vi "Receiver_Example - 2 Channel - Experiment_4.vi"() -> ()   [LabVIEW 2022 SP3]
panel:
  in  "Counter":dbl
  in  "State":i32
  out "CH0":bool
  out "CH1":bool
  out "iterationsIM":dbl
  out "High-Power Image 2":T1(plugin-control)
  out "High-Power Decoded message - CH0":string
  out "High-Power BER":T2(graph)
  in  "High-Power Window Size":dbl=15.0 format="%#_6p"
  in  "Low-Power Window Size - CH0":dbl=15.0 format="%#_6p"
  out "Low-Power BER - CH0":dbl(graph)
  out "Constellation Map":cluster{"Constellation":cdb[]}[](graph)
  in  "Tab Control":enum32{"USRP Parameters", "Rx Info", "BER"}(tab)
  in  "USRP ControledParameters":T3={"Active Antenna"="RX2", "Gain (dB)"=10.0, "Carrier Frequency"=2400000000.0, "IQ Rate"=2000000.0, "Active channels"="0,1"} {"IQ Rate" format="%#_6p"; "Carrier Frequency" format="%#_6p"; "Gain (dB)" format="%#_6f"}
  in  "Device selection":refnum<k15>="RIO0"
  in  "Trigger level":dbl=0.005 format="%f"
  out "CH0":T4
  out "CH1":T4
  out "SIG valid? - CH1":bool
  out "SIG valid? - CH0":bool
  out "Frequency offset - CH1":dbl
  out "Frequency offset - CH0":dbl
  out "Coerced Parameters":T5={"IQ Rate"=100000.0, "Carrier  Freq."=100000.0, "Gain"=0.0} {"Gain" format="%#_6f"; "Carrier  Freq." format="%#_6p"; "IQ Rate" format="%#_6p"}
  out "Error out":errorcluster
  in  "Expected message LP - CH0":string="Non Critical Data\nNon Critical Data\nNon Critical Data\nNon Critical Data\nNon Critical Data"
  in  "Expected message - CH1":string="Critical Dataaaaa\nCritical Dataaaaa\nCritical Dataaaaa\nCritical Dataaaaa\nCritical Dataaaaa"
  out "Expected message LP Detected CH0":string="Non Critical Data\nNon Critical Data\nNon Critical Data\nNon Critical Data\nNon Critical Data"
  out "Expected message HP Detected CH1":string="Non Critical Data\nNon Critical Data\nNon Critical Data\nNon Critical Data\nNon Critical Data"
  in  "Boolean":bool
  in  "Boolean 3":bool
  out "Expected message HP Detected CH0":string="Non Critical Data\nNon Critical Data\nNon Critical Data\nNon Critical Data\nNon Critical Data"
  in  "Expected message HP - CH0":string="Critical Dataaaaa\nCritical Dataaaaa\nCritical Dataaaaa\nCritical Dataaaaa\nCritical Dataaaaa"
  in  "Boolean 2":bool
  out "Inst. BER HP - CH0":dbl format="%#_4g"
  out "Acc. BER HP - CH0":dbl format="%#_4g"
  out "Acum. Err HP - CH0":dbl
  out "No. Bits HP - CH0":dbl
  out "Acc. BER LP - CH0":dbl format="%#_4g"
  out "Inst. BER - CH1":dbl format="%#_4g"
  out "Inst. BER LP - CH0":dbl format="%#_4g"
  out "No. Bits - CH1":dbl
  out "No. Bits LP - CH0":dbl
  out "Acum. Err - CH1":dbl
  out "Acum. Err LP - CH0":dbl
  in  "Record BER":bool
  in  "Refresh Button":bool
  out "Acc. BER - CH1":dbl format="%#_4g"
  in  "error in (no error)":errorcluster
  out "Decoded message - CH1":string
  out "Low-Power Decoded message - CH0":string
  # "OFDM Superposition Coded Receiver"
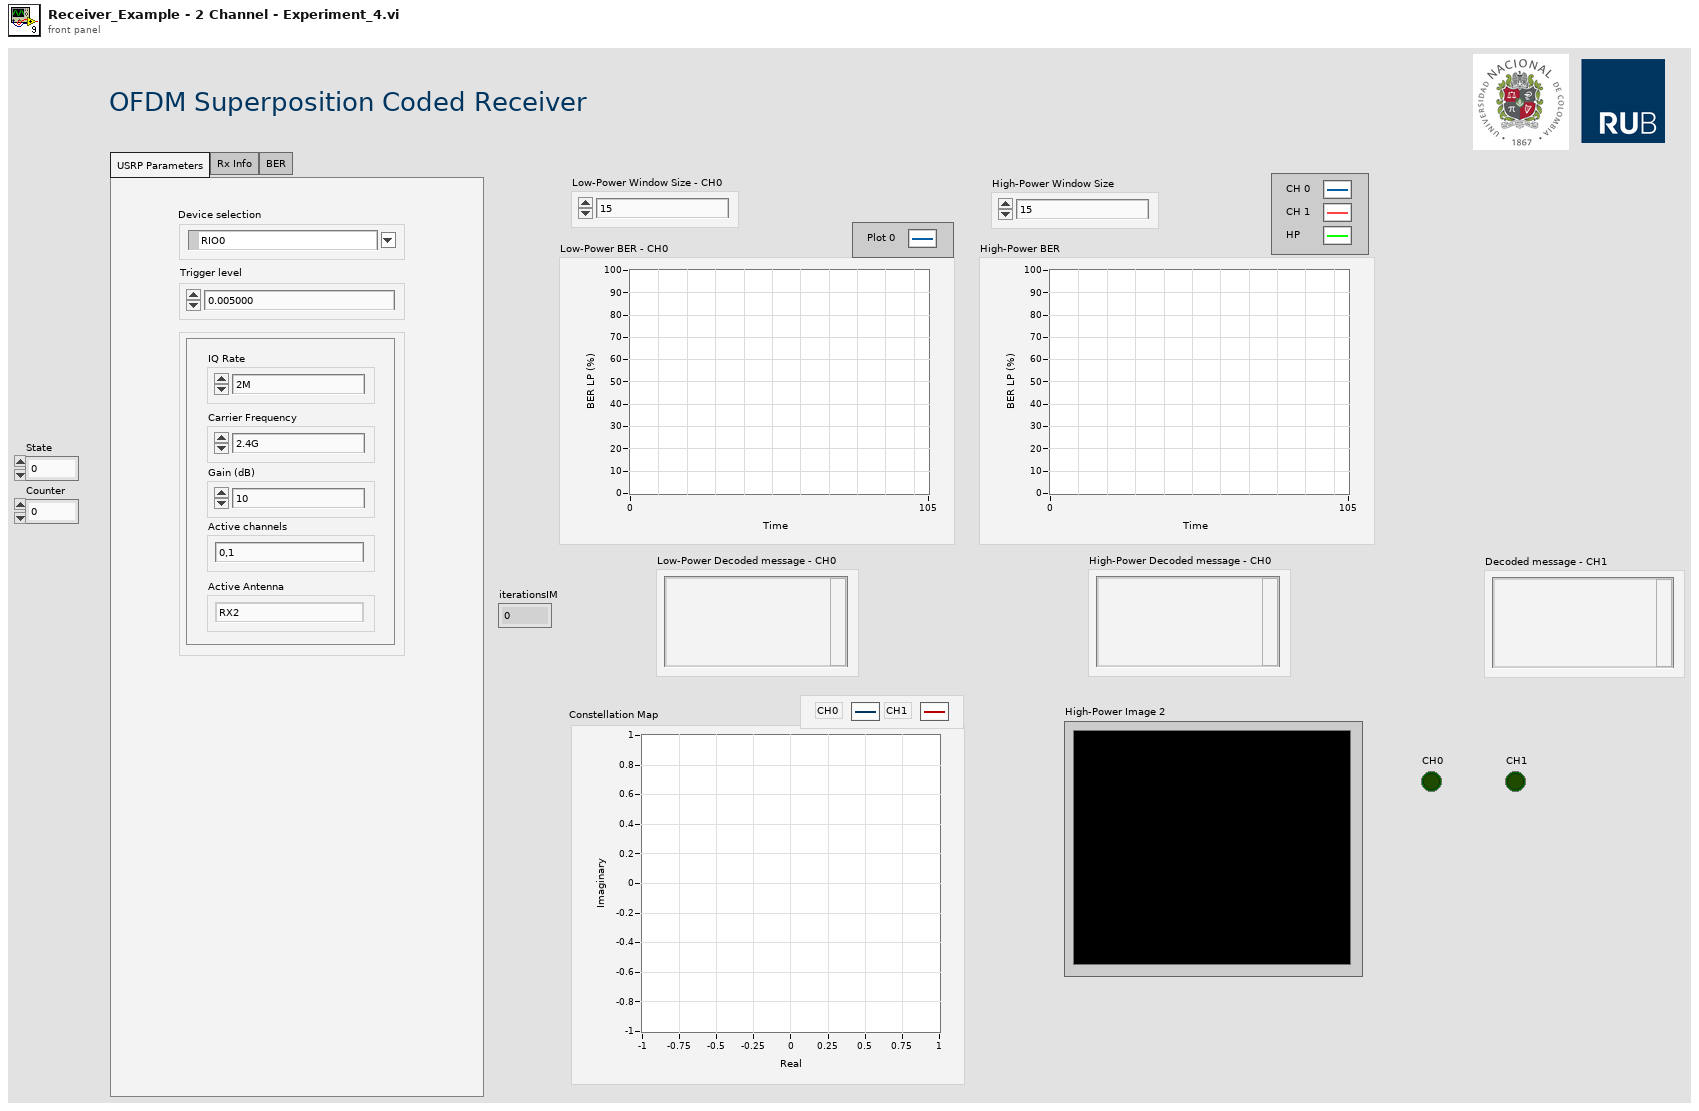
[diagram p1: front panel]
types:
  T1 = typedef "IMAQ Image.ctl" = refnum<image>
  T2 = cluster{"Graph Instantaneous BER":dbl, "Graph Instantaneous BER":dbl, "Inst. BER - CH1":dbl}
  T3 = cluster{"Active Antenna":string, "Gain (dB)":dbl, "Carrier Frequency":dbl, "IQ Rate":dbl, "Active channels":string}
  T4 = cluster{"Modulation type":enum16{"QPSK(4QAM)", "64QAM", "16QAM", "BPSK"}, "BCC rate (k/n)":enum16{"1/2", "2/3", "3/4"}}
  T5 = cluster{"IQ Rate":dbl, "Carrier  Freq.":dbl, "Gain":dbl}
  T6 = cluster{"coerced IQ rate":dbl, "coerced carrier frequency":dbl, "coerced gain":dbl}
  T7 = cluster{"Graph Instantaneous BER":dbl, "Graph Instantaneous BER":dbl, "Graph Instantaneous BER":dbl}
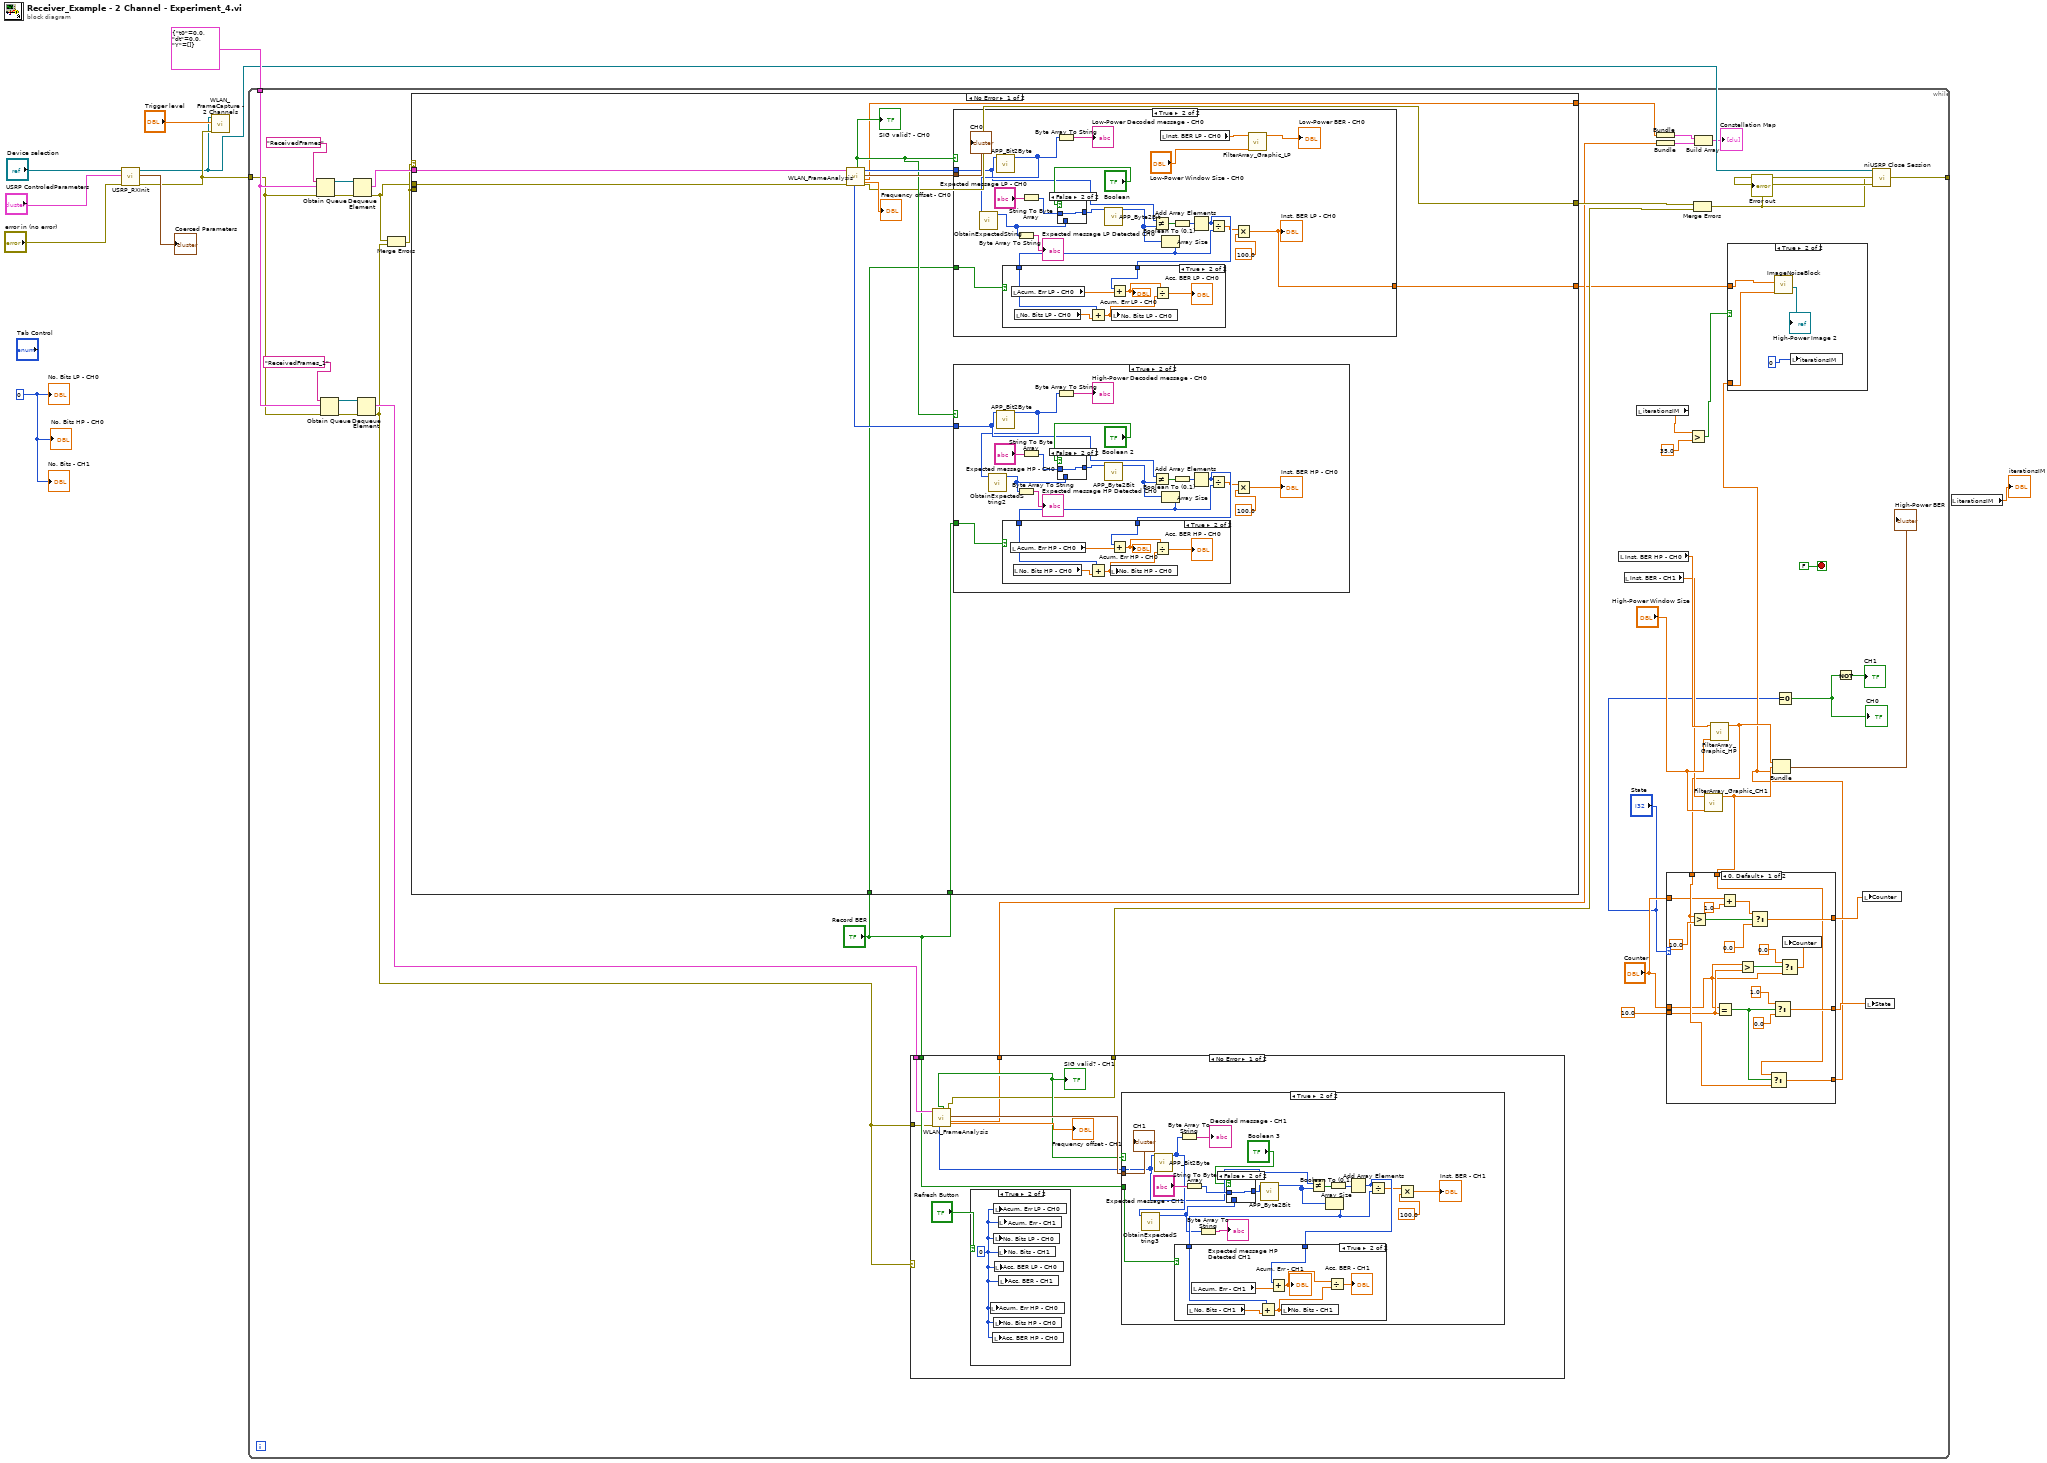
[diagram p0: block diagram]
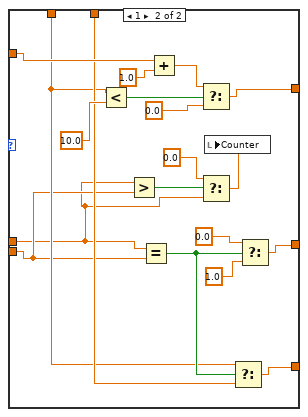
[diagram p2: hidden frame]
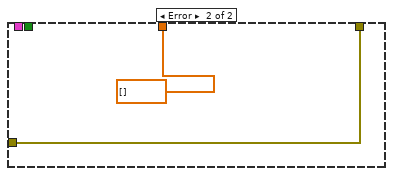
[diagram p7: hidden frame]
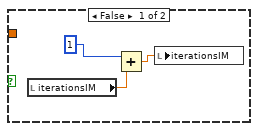
[diagram p8: hidden frame]
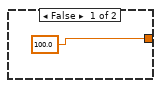
[diagram p12: hidden frame]
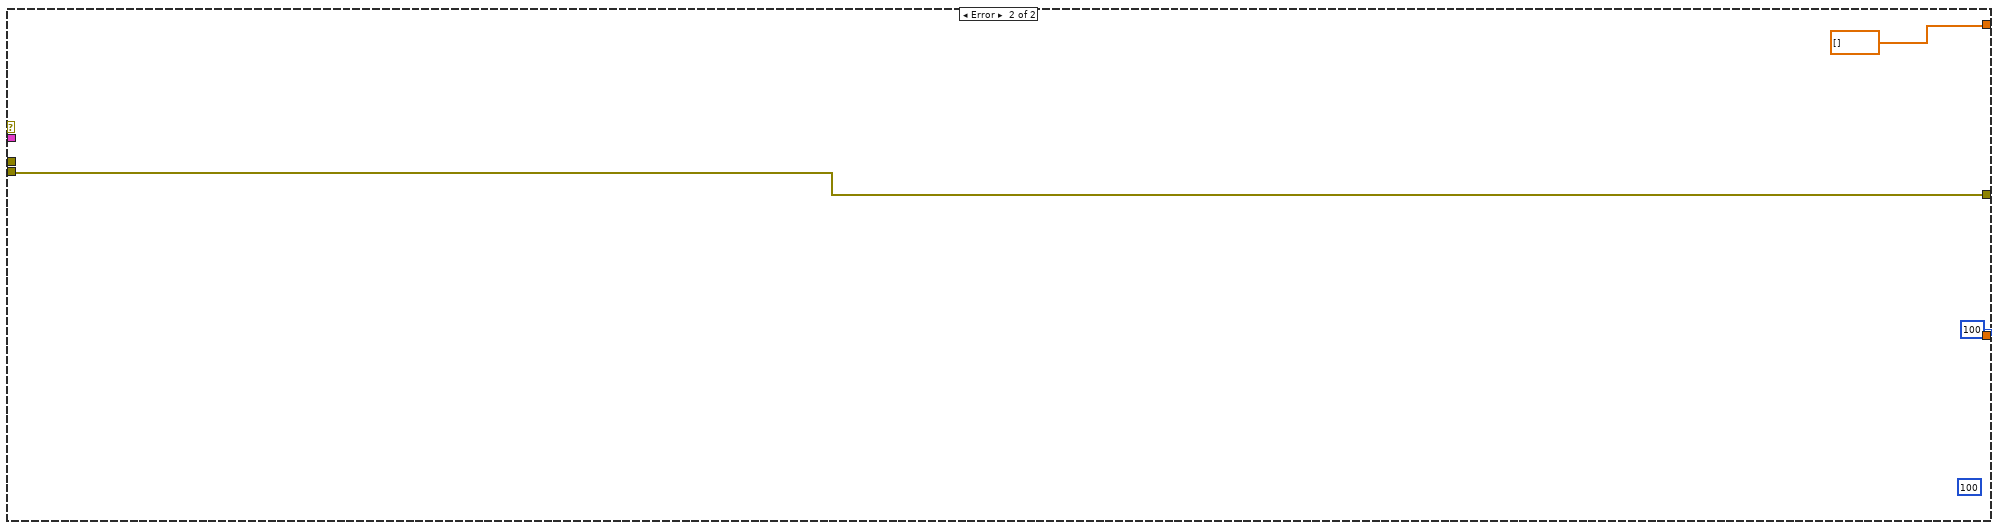
[diagram p15: hidden frame]
diagram:
  w2 = 0
  n1 = call "USRP_RXInit.vi"("device names"="Device selection", "USRP ControledParameters"="USRP ControledParameters", "error in (no error)"="error in (no error)") -> ("session handle out"=w5:refnum<k15>, "USRP CoercedParamters"=→"Coerced Parameters":T6, "error out"=w9:errorcluster)  [unwired: 5 in]
  n2 = call "WLAN_FrameCapture - 2 Channels.vi"("error in (no error)"=w9, "Trigger level"="Trigger level", "session handle"=w5) -> ()  [unwired: 8 in]
  n3 = while {
    tunnel: w9 -> [w44]
    tunnel: cluster{"t0":dbl, "dt":dbl, "Y":cdb[]} {"t0"=0.0, "dt"=0.0, "Y"=[]} ("data") -> [w45]
    tunnel: [w30] -> w6
    stop <- FALSE stop-if-true
    n4 = Obtain Queue(name (unnamed)="ReceivedFrames", element data type=w45, error in (no error)=w44) -> (queue out=w52:refnum<queue>, error out=w50:errorcluster)  [unwired: 2 in, 1 out]
    n5 = Obtain Queue(name (unnamed)="ReceivedFrames_1", element data type=w45, error in (no error)=w44) -> (queue out=w48:refnum<queue>, error out=w47:errorcluster)  [unwired: 2 in, 1 out]
    n6 = Dequeue Element(queue=w52, error in (no error)=w50) -> (element=w51:cluster{"t0":dbl, "dt":dbl, "Y":cdb[]}, error out=w41:errorcluster)  [unwired: 1 in, 2 out]
    n7 = Dequeue Element(queue=w48, error in (no error)=w47) -> (element=w33:cluster{"t0":dbl, "dt":dbl, "Y":cdb[]}, error out=w28:errorcluster)  [unwired: 1 in, 2 out]
    n8 = Merge Errors(w41, w28) -> (w42:errorcluster)
    n9 = case shown="No Error" w42 {
      tunnel: w51 -> [w147 _]
      tunnel: w42 -> [_ w211]
      tunnel: w41 -> [w144 _]
      tunnel: [w143 100] -> w26
      tunnel: [w142 dbl[] []] -> w34
      tunnel: [w141 w211] -> w32
      tunnel: "Record BER" -> [w140 _]
      tunnel: "Record BER" -> [w139 _]
      frame No Error {
        n10 = call "WLAN_FrameAnalysis.vi"("error in (no error)"=w144, "input cluster"=w147) -> ("error out"=w141:errorcluster, "Constellation"=w142:cdb[], "Modulation parameter"=w148:T4, "output bits"=w149:i8[], "Frequency offset"=→"Frequency offset - CH0":dbl, "SIG valid?"=w145:bool, "outputbitsHP"=w146:i8[])  [unwired: 3 in]
        "SIG valid? - CH0" <- w145
        n11 = case shown="True" w145 {
          tunnel: w149 -> [_ w181]
          tunnel: w148 -> [_ w199]
          tunnel: w139 -> [_ w195]
          tunnel: [100.0 w180] -> w143
          frame False {
          }
          frame True {
            n12 = call "APP_Bit2Byte.vi"("input bit stream"=w181) -> ("output byte stream"=w185:u8[])  [unwired: 10 in]
            n13 = call "ObtainExpectedString.vi"("Array"=w185) -> ("detectedMessage"=w182:i8[])  [unwired: 9 in]
            n14 = Byte Array To String(unsigned byte array=w182) -> (string=→"Expected message LP Detected CH0":string)
            n15 = String To Byte Array(string="Expected message LP - CH0") -> (unsigned byte array=w186:u8[])
            n16 = Byte Array To String(unsigned byte array=w185) -> (string=→"Low-Power Decoded message - CH0":string)
            n17 = case shown="False" "Boolean" {
              tunnel: [w201 w202] -> w188
              tunnel: w186 -> [_ w202]
              tunnel: w182 -> [w201 _]
              frame True {
              }
              frame False {
              }
            }
            n18 = call "APP_Byte2Bit.vi"("input byte stream"=w188) -> ("output bit stream"=w187:i8[])  [unwired: 10 in]
            n19 = Not Equal?(x=w181, y=w187) -> (x != y?=w197:bool[])
            n20 = local read "Inst. BER LP - CH0"() -> (w191:dbl)
            n21 = Array Size(array=w187) -> (size(s)=w194:i32)
            n22 = Boolean To (0,1)(Boolean=w197) -> (0, 1=w198:i16[])
            n23 = Add Array Elements(numeric array=w198) -> (sum=w193:i16)
            n24 = case shown="True" w195 {
              tunnel: w194 -> [_ w208]
              tunnel: w193 -> [_ w206]
              frame False {
              }
              frame True {
                n25 = local read "Acum. Err LP - CH0"() -> (w207:dbl)
                n26 = local read "No. Bits LP - CH0"() -> (w209:dbl)
                n27 = Add(x=w208, y=w209) -> (x+y=w205:dbl)
                n28 = Add(x=w206, y=w207) -> (x+y=w204:dbl)
                "Acum. Err LP - CH0" <- w204
                n29 = local write "No. Bits LP - CH0"(w205) -> ()
                n30 = Divide(x=w204, y=w205) -> (x/y=→"Acc. BER LP - CH0":dbl)
              }
            }
            n31 = Divide(x=w193, y=w194) -> (x/y=w190:dbl)
            n32 = Multiply(x=w190, y=100.0) -> (x*y=w180:dbl)
            "Inst. BER LP - CH0" <- w180
            n33 = call "FilterArray_Graphic_LP.vi"("Window Size"="Low-Power Window Size - CH0", "Instantaneous BER"=w191) -> ("Graph Instantaneous BER"=→"Low-Power BER - CH0":dbl)  [unwired: 4 in, 1 out]
            "CH0" <- w199
          }
        }
        n34 = case shown="True" w145 {
          tunnel: w146 -> [_ w154]
          tunnel: w140 -> [_ w164]
          frame False {
          }
          frame True {
            n35 = call "APP_Bit2Byte.vi"("input bit stream"=w154) -> ("output byte stream"=w153:u8[])  [unwired: 10 in]
            n36 = call "ObtainExpectedString2.vi"("Array"=w153) -> ("detectedMessage"=w152:i8[])  [unwired: 9 in]
            n37 = Byte Array To String(unsigned byte array=w152) -> (string=→"Expected message HP Detected CH0":string)
            n38 = String To Byte Array(string="Expected message HP - CH0") -> (unsigned byte array=w157:u8[])
            n39 = Byte Array To String(unsigned byte array=w153) -> (string=→"High-Power Decoded message - CH0":string)
            n40 = case shown="False" "Boolean 2" {
              tunnel: [w169 w170] -> w159
              tunnel: w157 -> [_ w170]
              tunnel: w152 -> [w169 _]
              frame True {
              }
              frame False {
              }
            }
            n41 = call "APP_Byte2Bit.vi"("input byte stream"=w159) -> ("output bit stream"=w158:i8[])  [unwired: 10 in]
            n42 = Not Equal?(x=w154, y=w158) -> (x != y?=w166:bool[])
            n43 = Array Size(array=w158) -> (size(s)=w163:i32)
            n44 = Boolean To (0,1)(Boolean=w166) -> (0, 1=w167:i16[])
            n45 = Add Array Elements(numeric array=w167) -> (sum=w162:i16)
            n46 = case shown="True" w164 {
              tunnel: w163 -> [_ w176]
              tunnel: w162 -> [_ w174]
              frame False {
              }
              frame True {
                n47 = local read "Acum. Err HP - CH0"() -> (w175:dbl)
                n48 = local read "No. Bits HP - CH0"() -> (w177:dbl)
                n49 = Add(x=w176, y=w177) -> (x+y=w173:dbl)
                n50 = local write "No. Bits HP - CH0"(w173) -> ()
                n51 = Add(x=w174, y=w175) -> (x+y=w172:dbl)
                "Acum. Err HP - CH0" <- w172
                n52 = Divide(x=w172, y=w173) -> (x/y=→"Acc. BER HP - CH0":dbl)
              }
            }
            n53 = Divide(x=w162, y=w163) -> (x/y=w161:dbl)
            n54 = Multiply(x=w161, y=100.0) -> (x*y=→"Inst. BER HP - CH0":dbl)
          }
        }
      }
      frame Error {
        (unwired) 100
      }
    }
    n55 = case shown="No Error" w28 {
      tunnel: w33 -> [w96 _]
      tunnel: "Record BER" -> [w94 _]
      tunnel: [w93 w131] -> w31
      tunnel: [w92 dbl[] []] -> w29
      tunnel: w28 -> [w91 w131]
      frame No Error {
        n56 = call "WLAN_FrameAnalysis.vi"("error in (no error)"=w91, "input cluster"=w96) -> ("error out"=w93:errorcluster, "Constellation"=w92:cdb[], "Modulation parameter"=w99:T4, "Frequency offset"=→"Frequency offset - CH1":dbl, "SIG valid?"=w95:bool, "outputbitsHP"=w97:i8[])  [unwired: 3 in, 1 out]
        "SIG valid? - CH1" <- w95
        n57 = case shown="True" "Refresh Button" {
          frame False {
          }
          frame True {
            w101 = 0
            n58 = local write "Acum. Err HP - CH0"(w101) -> ()
            n59 = local write "Acc. BER HP - CH0"(w101) -> ()
            n60 = local write "Acum. Err LP - CH0"(w101) -> ()
            n61 = local write "No. Bits LP - CH0"(w101) -> ()
            n62 = local write "No. Bits HP - CH0"(w101) -> ()
            n63 = local write "Acc. BER LP - CH0"(w101) -> ()
            n64 = local write "Acum. Err - CH1"(w101) -> ()
            n65 = local write "No. Bits - CH1"(w101) -> ()
            n66 = local write "Acc. BER - CH1"(w101) -> ()
          }
        }
        n67 = case shown="True" w95 {
          tunnel: w97 -> [_ w105]
          tunnel: w99 -> [_ w120]
          tunnel: w94 -> [_ w102]
          frame False {
          }
          frame True {
            n68 = call "APP_Bit2Byte.vi"("input bit stream"=w105) -> ("output byte stream"=w108:u8[])  [unwired: 10 in]
            n69 = call "ObtainExpectedString3.vi"("Array"=w108) -> ("detectedMessage"=w107:i8[])  [unwired: 9 in]
            n70 = Byte Array To String(unsigned byte array=w108) -> (string=→"Decoded message - CH1":string)
            n71 = String To Byte Array(string="Expected message - CH1") -> (unsigned byte array=w109:u8[])
            n72 = Byte Array To String(unsigned byte array=w107) -> (string=→"Expected message HP Detected CH1":string)
            n73 = case shown="False" "Boolean 3" {
              tunnel: [w121 w122] -> w111
              tunnel: w109 -> [_ w122]
              tunnel: w107 -> [w121 _]
              frame True {
              }
              frame False {
              }
            }
            n74 = call "APP_Byte2Bit.vi"("input byte stream"=w111) -> ("output bit stream"=w110:i8[])  [unwired: 10 in]
            n75 = Not Equal?(x=w105, y=w110) -> (x != y?=w117:bool[])
            n76 = Array Size(array=w110) -> (size(s)=w115:i32)
            n77 = Boolean To (0,1)(Boolean=w117) -> (0, 1=w118:i16[])
            n78 = Add Array Elements(numeric array=w118) -> (sum=w114:i16)
            n79 = case shown="True" w102 {
              tunnel: w115 -> [_ w128]
              tunnel: w114 -> [_ w126]
              frame False {
              }
              frame True {
                n80 = local read "No. Bits - CH1"() -> (w129:dbl)
                n81 = local read "Acum. Err - CH1"() -> (w127:dbl)
                n82 = Add(x=w128, y=w129) -> (x+y=w125:dbl)
                n83 = Add(x=w126, y=w127) -> (x+y=w124:dbl)
                "Acum. Err - CH1" <- w124
                n84 = local write "No. Bits - CH1"(w125) -> ()
                n85 = Divide(x=w124, y=w125) -> (x/y=→"Acc. BER - CH1":dbl)
              }
            }
            n86 = Divide(x=w114, y=w115) -> (x/y=w112:dbl)
            n87 = Multiply(x=w112, y=100.0) -> (x*y=→"Inst. BER - CH1":dbl)
            "CH1" <- w120
          }
        }
      }
      frame Error {
      }
    }
    n88 = local read "Inst. BER HP - CH0"() -> (w19:dbl)
    n89 = local read "Inst. BER - CH1"() -> (w18:dbl)
    n90 = local read "iterationsIM"() -> (w40:dbl)
    n91 = Bundle("Constellation"=w34) -> (w37:cluster{"Constellation":cdb[]})  [unwired: 1 in]
    n92 = Bundle("Constellation"=w29) -> (w36:cluster{"Constellation":cdb[]})  [unwired: 1 in]
    n93 = Greater?(x=w40, y=35.0) -> (0:w39:bool)
    n94 = Merge Errors(w32, w31) -> (w30:errorcluster)
    "Error out" <- w30
    n95 = Build Array(w37, w36) -> (→"Constellation Map":cluster{"Constellation":cdb[]}[])
    n96 = call "FilterArray_Graphic_CH1.vi"("Window Size"="High-Power Window Size", "Instantaneous BER"=w18) -> ("Graph Instantaneous BER"=w16:dbl)  [unwired: 4 in, 1 out]
    n97 = call "FilterArray_Graphic_HP.vi"("Window Size"="High-Power Window Size", "Instantaneous BER"=w19) -> ("Graph Instantaneous BER"=w17:dbl)  [unwired: 4 in, 1 out]
    n98 = case shown="0, Default" "State" {
      tunnel: "Counter" -> [w59 w79]
      tunnel: [w66 w82] -> w23
      tunnel: "Counter" -> [w54 w72]
      tunnel: [w63 w81] -> w22
      tunnel: [w61 w80] -> w15
      tunnel: w17 -> [w60 w77]
      tunnel: w16 -> [w58 w78]
      tunnel: 10.0 ("y") -> [w57 w73]
      frame 0, Default {
        n99 = Greater?(x=w60, y=10.0) -> (0:w67:bool)
        n100 = Equal?(x=w54, y=w57) -> (x = y?=w62:bool)
        n101 = Add(x=w59, y=1.0) -> (x+y=w69:dbl)
        n102 = Greater?(x=w54, y=w57) -> (0:w56:bool)
        n103 = Select(t=w69, s=w67, f=0.0) -> (s? t:f=w66:dbl)
        n104 = Select(t=w58, s=w62, f=w60) -> (s? t:f=w61:dbl)
        n105 = Select(t=1.0, s=w62, f=0.0) -> (s? t:f=w63:dbl)
        n106 = Select(t=0.0, s=w56, f=w54) -> (s? t:f=w53:dbl)
        n107 = local write "Counter"(w53) -> ()
      }
      frame 1 {
        n108 = Less?(x=w77, y=10.0) -> (x < y?=w83:bool)
        n109 = Greater?(x=w72, y=w73) -> (0:w75:bool)
        n110 = Equal?(x=w72, y=w73) -> (x = y?=w85:bool)
        n111 = Add(x=w79, y=1.0) -> (x+y=w89:dbl)
        n112 = Select(t=w89, s=w83, f=0.0) -> (s? t:f=w82:dbl)
        n113 = Select(t=0.0, s=w75, f=w72) -> (s? t:f=w76:dbl)
        n114 = local write "Counter"(w76) -> ()
        n115 = Select(t=w77, s=w85, f=w78) -> (s? t:f=w80:dbl)
        n116 = Select(t=0.0, s=w85, f=1.0) -> (s? t:f=w81:dbl)
      }
    }
    n117 = case shown="True" w39 {
      tunnel: w15 -> [_ w138]
      tunnel: w26 -> [_ w135]
      frame False {
        n118 = local read "iterationsIM"() -> (w134:dbl)
        n119 = Add(x=1, y=w134) -> (x+y=w133:dbl)
        n120 = local write "iterationsIM"(w133) -> ()
      }
      frame True {
        n121 = call "ImageNoiseBlock.vi"("BERLP"=w135, "BERHP"=w138) -> ("High-Power Image"=→"High-Power Image 2":T1)  [unwired: 8 in]
        n122 = local write "iterationsIM"(0) -> ()
      }
    }
    n123 = Bundle("Graph Instantaneous BER"=w17, "Graph Instantaneous BER"=w16, "Graph Instantaneous BER"=w15) -> (→"High-Power BER":T7)  [unwired: 1 in]
    n124 = Equal To 0?(x="State") -> (x = 0?=w12:bool)
    "CH0" <- w12
    n125 = Not(x=w12) -> (.not. x?=→"CH1":bool)
    n126 = local write "Counter"(w23) -> ()
    n127 = local write "State"(w22) -> ()
  }
  n128 = call <instrlib>:"niUSRP Close Session.vi"("session handle"=w5, "error in (no error)"=w6) -> ()  [unwired: 13 in, 1 out]
  n129 = local read "iterationsIM"() -> (→"iterationsIM":dbl)
  "No. Bits LP - CH0" <- w2
  "No. Bits - CH1" <- w2
  "No. Bits HP - CH0" <- w2
